vi "确定需要读取的参数个数.vi"(5 "Cmd":string) -> (1 "Cmd":i32=31, 2 "# parameters":i32=31)   [LabVIEW 2013]
doc: "此函数根据命令字的不同，查找预先定义好的每种命令对应的返回值的长度，用于返回值的读取。"
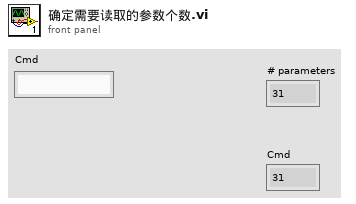
[diagram p1: front panel]
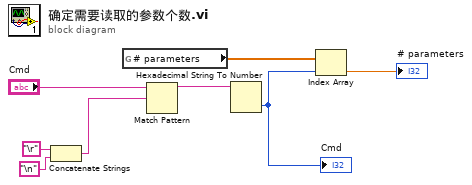
[diagram p0: block diagram]
diagram:
  n1 = Concatenate Strings("\r", "\n") -> (w6:string)
  n2 = global read "各个命令对应的读取次数.vi" "# parameters"() -> (w3:dbl[])
  n3 = Match Pattern(string="Cmd", regular expression=w6) -> (before substring=w4:string)  [unwired: 1 in, 3 out]
  n4 = Hexadecimal String To Number(string=w4) -> (number=w1:u32)  [unwired: 2 in, 1 out]
  "Cmd" <- w1
  n5 = Index Array(array=w3, index=w1) -> (element=→"# parameters":dbl)
